vi "File path.vi"(0 "folder name":string, 1 "file name":string, 2 "pattern":string, 3 "error in (no error)":errorcluster) -> (4 "root path":path, 5 "build path":path, 6 "directory path":path, 7 "File path":path, 8 "error out":errorcluster)   [LabVIEW 2010]
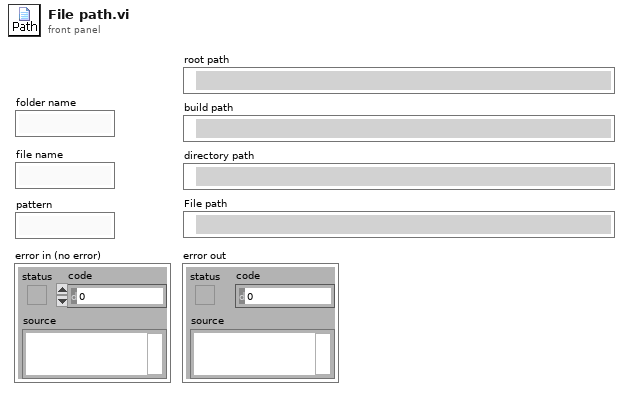
[diagram p1: front panel]
types:
  T1 = enum32{"invalid app kind", "Development System", "Run Time System", "Student Edition", "Embedded LabVIEW", "Evaluation", "Custom"}
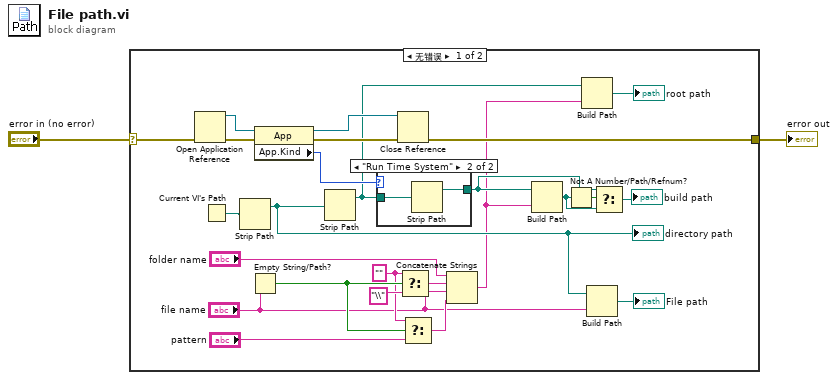
[diagram p0: block diagram]
diagram:
  n1 = case shown="无错误" "error in (no error)" {
    selector: "error in (no error)" -> [w14 w31]
    tunnel: [w13 w31] -> w1
    frame No Error {
      w11 = ""
      n2 = Open Application Reference(8:w14) -> (0:w25:errorcluster, 3:w24:refnum<vi>)  [unwired: 3 in]
      n3 = Current VI's Path() -> (path=w27:path)
      n4 = Strip Path(path=w27) -> (stripped path=w8:path)  [unwired: 1 out]
      "directory path" <- w8
      n5 = Empty String/Path?(string/path="file name") -> (empty?=w12:bool)
      n6 = property class="App"(reference=w24, error in=w25) -> (reference out=w22:refnum<vi>, error out=w23:errorcluster, "App.Kind"=w26:T1)
      n7 = Strip Path(path=w8) -> (stripped path=w4:path)  [unwired: 1 out]
      n8 = case shown="\"Run Time System\"" w26 {
        tunnel: w4 -> [w28 w30]
        tunnel: [w28 w29] -> w17
        frame "Development System", Default {
        }
        frame "Run Time System" {
          n9 = Strip Path(path=w30) -> (stripped path=w29:path)  [unwired: 1 out]
        }
      }
      n10 = Close Reference(reference=w22, error in (no error)=w23) -> (error out=w13:errorcluster)
      n11 = Select(t=w11, s=w12, f="\\") -> (s? t:f=w19:string)
      n12 = Select(t=w11, s=w12, f="pattern") -> (s? t:f=w9:string)
      n13 = Concatenate Strings("folder name", w19, "file name", w9) -> (w3:string)
      n14 = Build Path(base path=w17, name or relative path=w3) -> (appended path=w16:path)
      n15 = Not A Number/Path/Refnum?(number/path/refnum=w16) -> (NaN/Path/Refnum?=w20:bool)
      n16 = Build Path(base path=w4, name or relative path=w3) -> (appended path=→"root path":path)
      n17 = Build Path(base path=w8, name or relative path="file name") -> (appended path=→"File path":path)
      n18 = Select(t=w17, s=w20, f=w16) -> (s? t:f=→"build path":path)
    }
    frame Error {
    }
  }
  "error out" <- w1
